vi "Get Values Array.vi"(8 "error in (no error)":errorcluster, 11 "Simulated VeriStand Engine in":refnum<class "Simulated VeriStand Engine.lvclass">) -> (0 "error out":errorcluster, 2 "Values Array":dbl[](array[numeric]), 3 "Simulated VeriStand Engine out":refnum<class "Simulated VeriStand Engine.lvclass">)   [LabVIEW 2016, in "Simulated VeriStand Engine.lvclass"]
uses:
  Simulated VeriStand Engine.lvclass
  Simulated VeriStand Engine.lvclass/Simulated VeriStand Engine.ctl
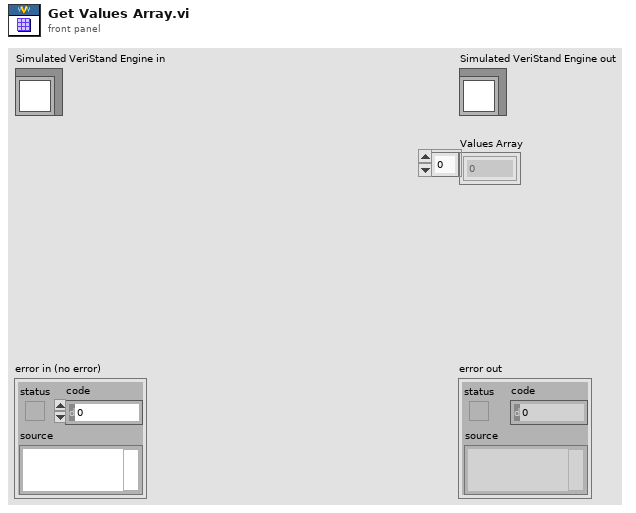
[diagram p1: front panel]
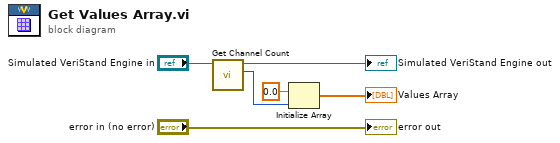
[diagram p0: block diagram]
diagram:
  n1 = call "Get Channel Count.vi"("Simulated VeriStand Engine in"="Simulated VeriStand Engine in") -> ("Channel Count"=w2:u32, "Simulated VeriStand Engine out"=→"Simulated VeriStand Engine out":refnum<class "Simulated VeriStand Engine.lvclass">)  [unwired: 8 in, 1 out]
  n2 = Initialize Array(0.0 ("element"), w2) -> (→"Values Array":dbl[])
  "error out" <- "error in (no error)"
